vi "Active Line Name.vi"(8 "error in":errorcluster, 11 "Data Grid in":refnum<class "Data Grid.lvclass">) -> (0 "error out":errorcluster, 2 "Active Line Name":string, 3 "Data Grid out":refnum<class "Data Grid.lvclass">)   [LabVIEW 2013, in "Table Manager.lvlib" / "Data Grid.lvclass"]
uses:
  Data Grid.lvclass
  Data Grid.lvclass/Data Grid.ctl
  Read DataGridView.vi
  Write DataGridView.vi
  Table Manager/Table Manager.lvclass
  <vilib>/LabVIEW DataGridView/source/DataGridView/DataGridView.lvclass
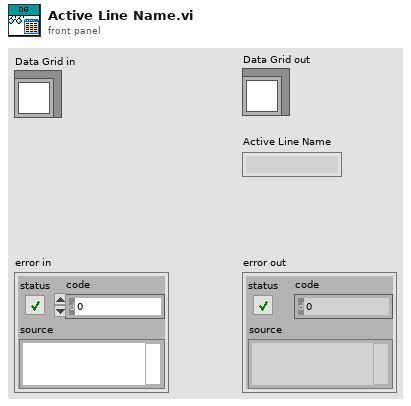
[diagram p1: front panel]
types:
  T1 = typedef "Table Manager.lvlib/Table Manager.lvclass/object ref.ctl" = cluster{"engine":refnum<data-value>, "Node Ref":refnum<data-value>}
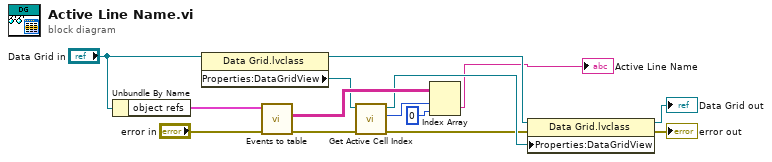
[diagram p0: block diagram]
diagram:
  n1 = Unbundle By Name("Data Grid in") -> ("object refs"=w7:T1)
  n2 = property class="Data Grid.lvclass"(reference="Data Grid in") -> (reference out=w9:refnum<class "Data Grid.lvclass">, "Properties:DataGridView"=w11:refnum<class "DataGridView.lvclass">)  [unwired: 1 in, 1 out]
  n3 = call "Events to table.vi"("error in (no error)"="error in", "object ref in"=w7) -> ("error out"=w12:errorcluster, "table"=w14:string[][])  [unwired: 7 in, 1 out]
  n4 = call <vilib>:"Get Active Cell Index.vi"("error in (no error)"=w12, "DataGridView in"=w11) -> ("error out"=w1:errorcluster, "RowIndex"=w8:i32, "DataGridView out"=w10:refnum<class "DataGridView.lvclass">)  [unwired: 6 in, 1 out]
  n5 = Index Array(array=w14, index (row)=w8, index (col)=0 ("disabled index (col)")) -> (element=→"Active Line Name":string)
  n6 = property class="Data Grid.lvclass"(reference=w9, error in=w1, "Properties:DataGridView"=w10) -> (reference out=→"Data Grid out":refnum<class "Data Grid.lvclass">, error out=→"error out":errorcluster)
